vi "Solution Data Extractor.vi"(8 "Error In":errorcluster, 9 "Solution Data":variant[][](array[variant])=[[variant]], 10 "Solution Label":string, 11 "Author ID":i32) -> (0 "Error Out":errorcluster, 2 "Exists?":bool, 3 "Solution Information":T1)   [LabVIEW 2020]
uses:
  <vilib>/addons/database/_DB Variant To Data/Database Variant To Data.xnode
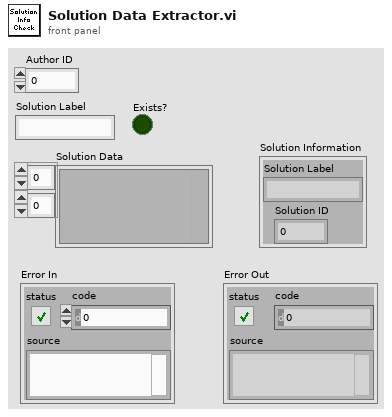
[diagram p1: front panel]
types:
  T1 = cluster{"Solution Label":string, "Solution ID":i32}
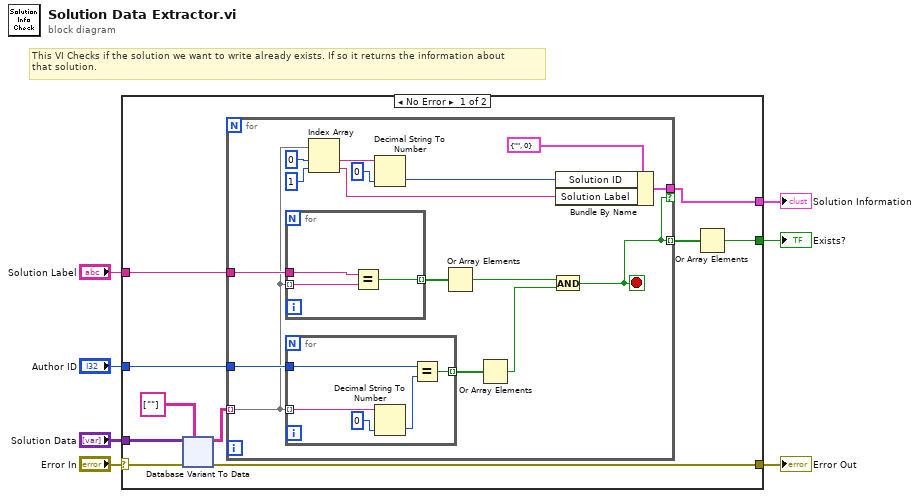
[diagram p0: block diagram]
diagram:
  # "This VI Checks if the solution we want to write already exists. If so it returns the information about\nthat solution."
  n1 = case shown="No Error" "Error In" {
    selector: "Error In" -> [w13 w86]
    tunnel: "Solution Data" -> [w14 _]
    tunnel: "Solution Label" -> [w12 _]
    tunnel: [w10 _] -> w4
    tunnel: [w11 w86] -> w3
    tunnel: [w8 _] -> w2
    tunnel: "Author ID" -> [w9 _]
    frame No Error {
      n2 = xnode "Database Variant To Data"("database variant"=w14, "error in (no error)"=w13, "type"=string[][] [[""]] ("columns")) -> ("data"=w15:string[][], "error out"=w11:errorcluster)
      n3 = for {
        tunnel: w15 -> [w22] mode=indexing
        tunnel: w12 -> [w33]
        tunnel: [w18] -> w16 mode=indexing
        tunnel: [w24] -> w8 if=w18
        tunnel: w9 -> [w23]
        stop <- w18 stop-if-true
        n4 = for {
          tunnel: w22 -> [w40] mode=indexing
          tunnel: w33 -> [w41]
          tunnel: [w39] -> w32 mode=indexing
          n5 = Equal?(x=w41, y=w40) -> (x = y?=w39:bool)
        }
        n6 = for {
          tunnel: w22 -> [w35] mode=indexing
          tunnel: w23 -> [w38]
          tunnel: [w37] -> w21 mode=indexing
          n7 = Decimal String To Number(string=w35, default (0L)=0 ("default (0 I32)")) -> (number=w34:i32)  [unwired: 1 in, 1 out]
          n8 = Equal?(x=w38, y=w34) -> (x = y?=w37:bool)
        }
        n9 = Index Array(array=w22, index #1=0 ("index"), index #2=1 ("index")) -> (element #1=w29:string, element #2=w26:string)
        n10 = Decimal String To Number(string=w29, default (0L)=0 ("default (0 I32)")) -> (number=w25:i32)  [unwired: 1 in, 1 out]
        n11 = Or Array Elements(Boolean array=w32) -> (logical OR=w20:bool)
        n12 = Or Array Elements(Boolean array=w21) -> (logical OR=w19:bool)
        n13 = And(x=w20, y=w19) -> (x .and. y?=w18:bool)
        n14 = Bundle By Name(cluster=T1 {"Solution Label"="", "Solution ID"=0} ("output cluster"), "Solution ID"=w25, "Solution Label"=w26) -> (w24:T1)
      }
      n15 = Or Array Elements(Boolean array=w16) -> (logical OR=w10:bool)
    }
    frame Error {
    }
  }
  "Exists?" <- w4
  "Error Out" <- w3
  "Solution Information" <- w2
